vi "selection sort.vi"(11 "Array in":dbl[](array[numeric])) -> (2 "Waveform Graph":dbl[](graph), 3 "Array out":dbl[](array[numeric]))   [LabVIEW 2014]
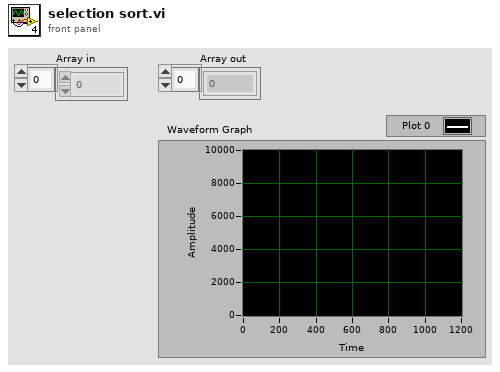
[diagram p1: front panel]
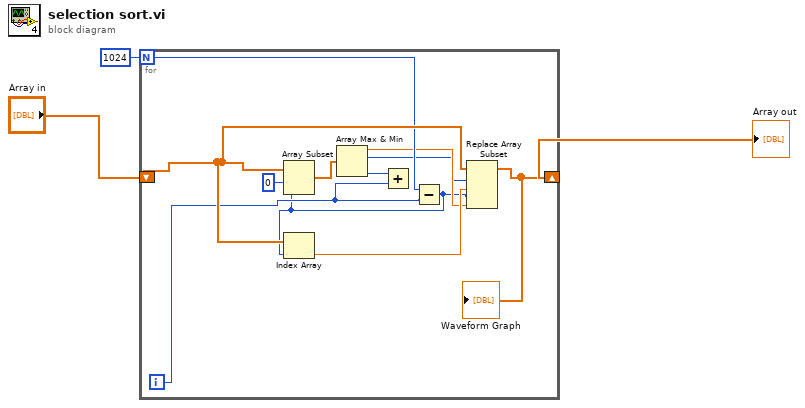
[diagram p0: block diagram]
diagram:
  n1 = for {
    N: 1024 -> [w9]
    shift-right: [w10] -> w3
    shift-left: "Array in" -> [w11]
    i -> [w6]
    n2 = Subtract(x=w9, y=w6) -> (x-y=w4:i32)
    n3 = Array Subset(array=w11, index=0, length=w4) -> (w14:dbl[])
    n4 = Index Array(array=w11, index=w4) -> (element=w12:dbl)
    n5 = Array Max & Min(array=w14) -> (max value=w8:dbl, max index (indices)=w7:i32, min index (indices)=w13:i32)  [unwired: 1 out]
    n6 = Add(x=w13, y=w6) -> ()  [unwired: 1 out]
    n7 = Replace Array Subset(array=w11, new element #1=w12, index #1=w7, new element #2=w8, index #2=w4) -> (w10:dbl[])
    "Waveform Graph" <- w10
  }
  "Array out" <- w3
